vi "String.vi"(0 "Amount":fxp<+,8,0>, 4 "S/R":fxp<+,16,0>, 5 "1/Decay":fxp<+,16,0>, 6 "Sustain":fxp<+,16,0>, 7 "1/Attack":fxp<+,16,0>, 8 "Gate":bool, 9 "LFO":fxp<+/-,8,8>, 10 "M":fxp<+,32,32>, 11 "Trigger":bool) -> (3 "String Out":fxp<+/-,8,8>)   [LabVIEW 2015]
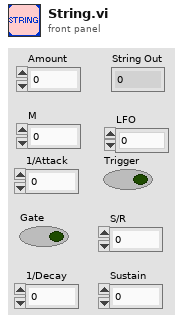
[diagram p1: front panel]
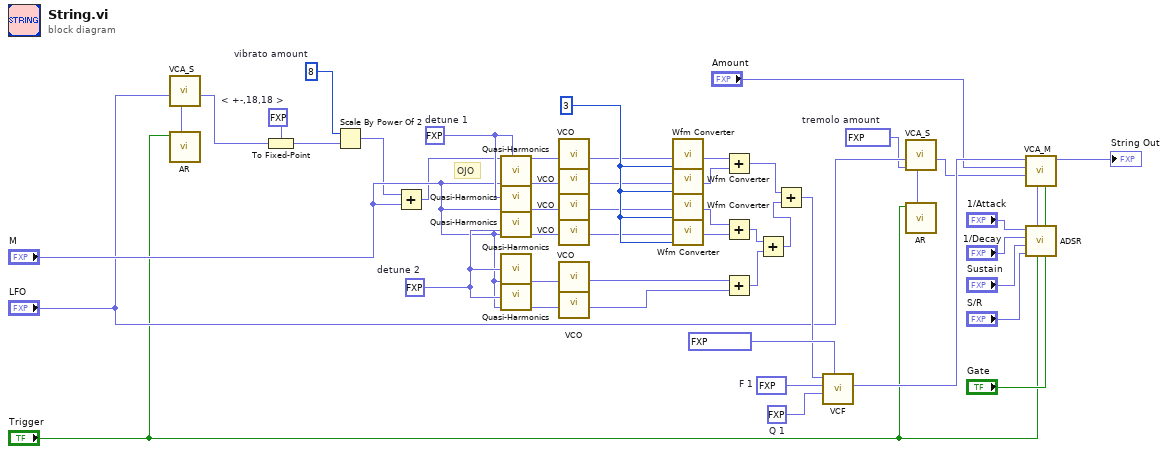
[diagram p0: block diagram]
diagram:
  w37 = u8 3 ("select")
  w4 = fxp<+,8,0> 0.28125  # tremolo amount
  w24 = fxp<+/-,18,18> 1.0  # Q 1
  w23 = fxp<+/-,18,18> 2300.0  # F 1
  w48 = fxp<+,8,3> 1.0  # detune 1
  w49 = fxp<+,8,3> 2.0  # detune 2
  w9 = i16 8  # vibrato amount
  w11 = fxp<+/-,18,18> 0.0  # < +-,18,18 >
  # "OJO"
  n1 = call "AR.vi"("Trigger"="Trigger") -> ("Sample Out"=w1:fxp<+,8,0>)  [unwired: 10 in]
  n2 = call "VCA_S.vi"("EG"=w1, "Sample In"="LFO") -> ("Sample Out"=w13:fxp<+/-,8,8>)  [unwired: 9 in]
  n3 = To Fixed-Point(fixed-point type=w11, number=w13) -> (fixed-point=w10:fxp<+/-,18,18>)
  n4 = Scale By Power Of 2(n=w9, x=w10) -> (x*2^n=w12:fxp<+/-,18,18>)
  n5 = Add(x=w12, y="M") -> (x+y=w8:fxp<+,32,32>)
  n6 = call "Quasi-Harmonics.vi"("Relative Freq"=w48, "1st partial"="M") -> ("Result Partial"=w34:fxp<+,32,32>)  [unwired: 9 in]
  n7 = call "Quasi-Harmonics.vi"("Relative Freq"=w48, "1st partial"="M") -> ("Result Partial"=w35:fxp<+,32,32>)  [unwired: 9 in]
  n8 = call "Quasi-Harmonics.vi"("Relative Freq"=w49, "1st partial"="M") -> ("Result Partial"=w36:fxp<+,32,32>)  [unwired: 9 in]
  n9 = call "Quasi-Harmonics.vi"("Relative Freq"=w49, "1st partial"="M") -> ("Result Partial"=w39:fxp<+,32,32>)  [unwired: 9 in]
  n10 = call "Quasi-Harmonics.vi"("Relative Freq"=w49, "1st partial"="M") -> ("Result Partial"=w38:fxp<+,32,32>)  [unwired: 9 in]
  n11 = call "VCO.vi"("M"=w8) -> ("Sine Sample"=w14:fxp<+/-,8,8>)  [unwired: 10 in]
  n12 = call "VCO.vi"("M"=w34) -> ("Sine Sample"=w25:fxp<+/-,8,8>)  [unwired: 10 in]
  n13 = call "VCO.vi"("M"=w35) -> ("Sine Sample"=w26:fxp<+/-,8,8>)  [unwired: 10 in]
  n14 = call "VCO.vi"("M"=w36) -> ("Sine Sample"=w27:fxp<+/-,8,8>)  [unwired: 10 in]
  n15 = call "VCO.vi"("M"=w39) -> ("Sine Sample"=w43:fxp<+/-,8,8>)  [unwired: 10 in]
  n16 = call "VCO.vi"("M"=w38) -> ("Sine Sample"=w44:fxp<+/-,8,8>)  [unwired: 10 in]
  n17 = call "Wfm Converter.vi"("Select"=w37, "Sample In"=w14) -> ("Sample Out"=w28:fxp<+/-,8,8>)  [unwired: 9 in]
  n18 = call "Wfm Converter.vi"("Select"=w37, "Sample In"=w25) -> ("Sample Out"=w29:fxp<+/-,8,8>)  [unwired: 9 in]
  n19 = call "Wfm Converter.vi"("Select"=w37, "Sample In"=w26) -> ("Sample Out"=w30:fxp<+/-,8,8>)  [unwired: 9 in]
  n20 = call "Wfm Converter.vi"("Select"=w37, "Sample In"=w27) -> ("Sample Out"=w31:fxp<+/-,8,8>)  [unwired: 9 in]
  n21 = Add(x=w28, y=w29) -> (x+y=w32:fxp<+/-,8,8>)
  n22 = Add(x=w30, y=w31) -> (x+y=w40:fxp<+/-,8,8>)
  n23 = Add(x=w43, y=w44) -> (x+y=w41:fxp<+/-,8,8>)
  n24 = Add(x=w40, y=w41) -> (x+y=w42:fxp<+/-,8,8>)
  n25 = Add(x=w32, y=w42) -> (x+y=w33:fxp<+/-,8,8>)
  n26 = call "VCF.vi"("Amount"=fxp<+,8,0> 0.99609375, "Q1"=w24, "F1"=w23, "Sample In"=w33) -> ("LP Out"=w46:fxp<+/-,8,8>)  [unwired: 5 in, 2 out]
  n27 = call "AR.vi"("Trigger"="Trigger") -> ("Sample Out"=w3:fxp<+,8,0>)  [unwired: 10 in]
  n28 = call "VCA_S.vi"("EG"=w3, "Amount"=w4, "Sample In"="LFO") -> ("Sample Out"=w15:fxp<+/-,8,8>)  [unwired: 8 in]
  n29 = call "ADSR.vi"("Gate"="Gate", "Trigger"="Trigger", "S/R"="S/R", "Sustain"="Sustain", "1/Decay"="1/Decay", "1/Attack"="1/Attack") -> ("Amount?"=w5:bool, "Sample Out"=w21:fxp<+,8,0>)  [unwired: 4 in]
  n30 = call "VCA_M.vi"("Amount?"=w5, "EG"=w21, "LFO"=w15, "Amount"="Amount", "Sample In"=w46) -> ("Sample Out"=→"String Out":fxp<+/-,8,8>)  [unwired: 6 in]
